vi "AR-AI-create.vi"(8 "error in":errorcluster, 11 "lines":tag="Dev1/ai0:3") -> (0 "error out":errorcluster, 3 "AI task out":refnum<k21>)   [LabVIEW 2021]
uses:
  <vilib>/DAQmx/create/channels.llb/DAQmx Create Channel (AI-Voltage-Basic).vi
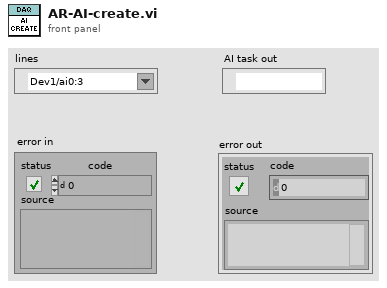
[diagram p1: front panel]
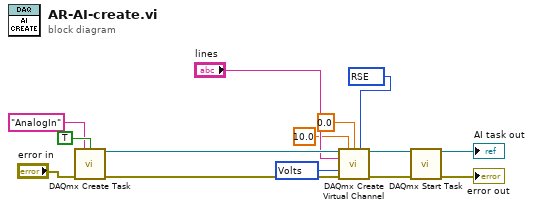
[diagram p0: block diagram]
diagram:
  w1 = 10348 items=["Volts"=10348, "From Custom Scale"=10065] ("units")
  w5 = 10083 items=["Default"=-1, "RSE"=10083, "NRSE"=10078, "Differential"=10106, "Pseudodifferential"=12529] ("input terminal configuration")
  n1 = call <vilib>:"DAQmx Create Task.vi"("new task name"="AnalogIn", "auto cleanup"=TRUE, "error in"="error in") -> ("task out"=w11:refnum<k21>, "error out"=w2:errorcluster)  [unwired: 11 in]
  n2 = call-poly <vilib>:"DAQmx Create Virtual Channel.vi"("task in"=w11, "maximum value"=10.0, "minimum value"=0.0, "input terminal configuration"=w5, "physical channels"="lines", "units"=w1, "error in"=w2) -> ("task out"=w10:refnum<k21>, "error out"=w12:errorcluster)  [unwired: 7 in]
  n3 = call <vilib>:"DAQmx Start Task.vi"("task/channels in"=w10, "error in"=w12) -> ("task out"=→"AI task out":refnum<k21>, "error out"=→"error out":errorcluster)  [unwired: 12 in]
